vi "Stack_holderwise_total_bd_count_&_duration.vi"(0 "Refnum in":T1, 1 "BREAKDOWN_STK_HOLD_ID":i32=1, 2 "condition":string="Where BREAKDOWN_DATE between '%s'and '%s' and BREAKDOWN_STK_HOLD_ID ='%d'  ", 5 "Form Date":timestamp, 7 "Array":string[](array[string]), 9 "To Date":timestamp, 11 "error in (no error)":errorcluster, 12 "STATION_ID_CID_TRIGGER":i32, 13 "Shift":string(combo), 14 "tabel":string[](array[string])=["STATION_1_LOG_HISTORY", "STATION_2_LOG_HISTORY", "STATION_3_LOG_HISTORY", "STATION_4_LOG_HISTORY", "STATION_5_LOG_HISTORY", "STATION_6_LOG_HISTORY"]) -> (4 "Refnum out":T1, 6 "Count out":string[](array[string]), 10 "appended array":dbl[](array[numeric]), 15 "error out":errorcluster)   [LabVIEW 2017]
uses:
  <vilib>/addons/database/Connection.llb/Conn ObjectReference.ctl
  <vilib>/addons/database/NI_Database_API.lvlib
panel:
  out "Elements Found out":string[](array[string])
  out "Table":string[][](array[string])
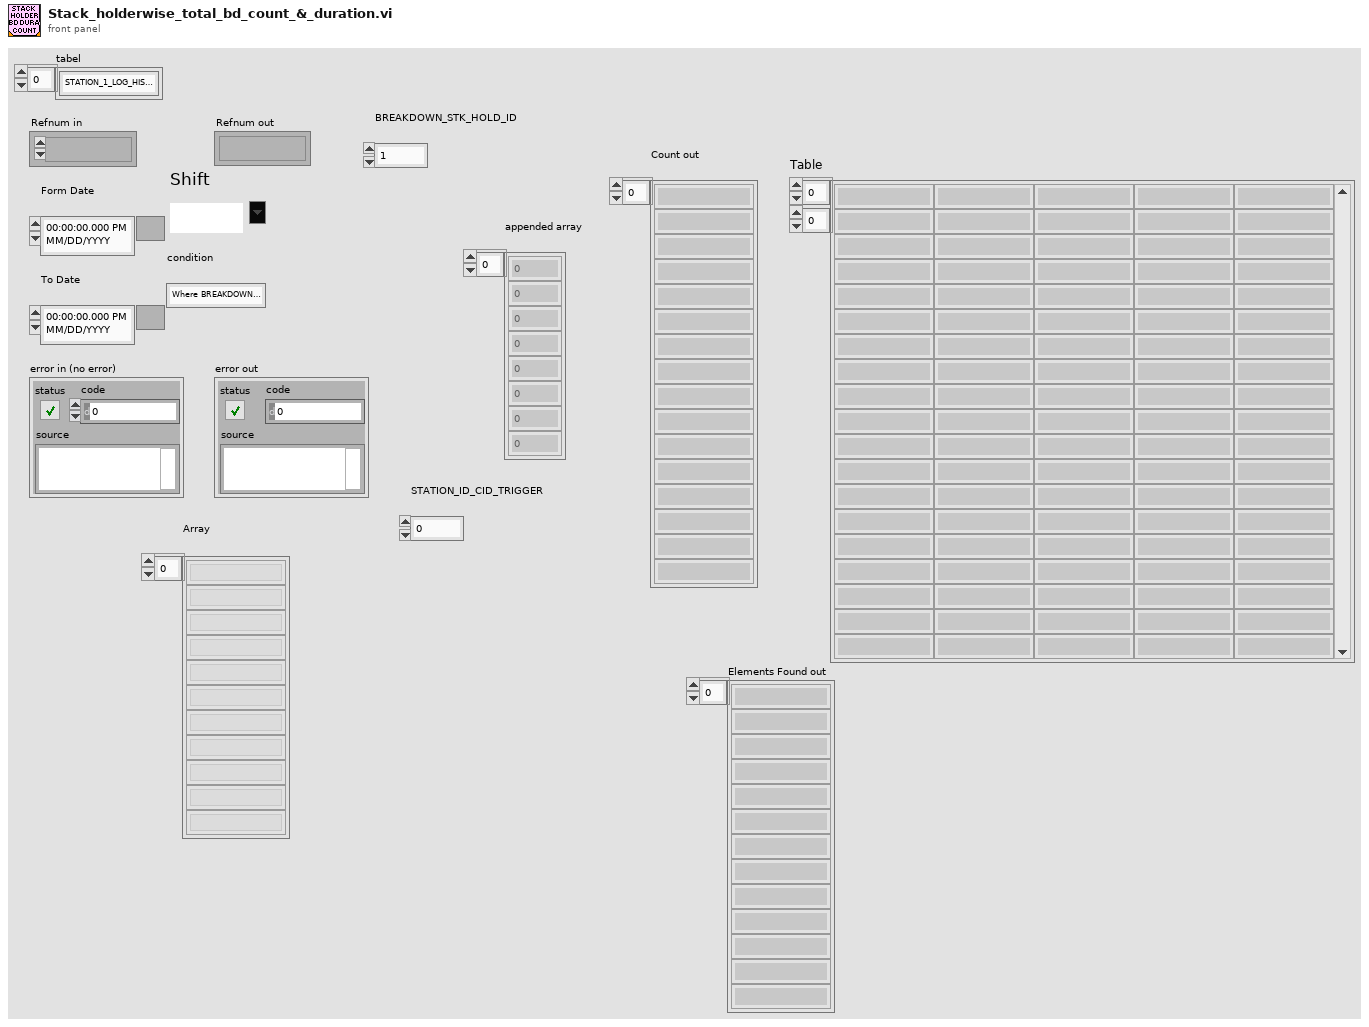
[diagram p1: front panel]
types:
  T1 = typedef "NI_Database_API.lvlib/Conn ObjectReference.ctl" = refnum<k1>
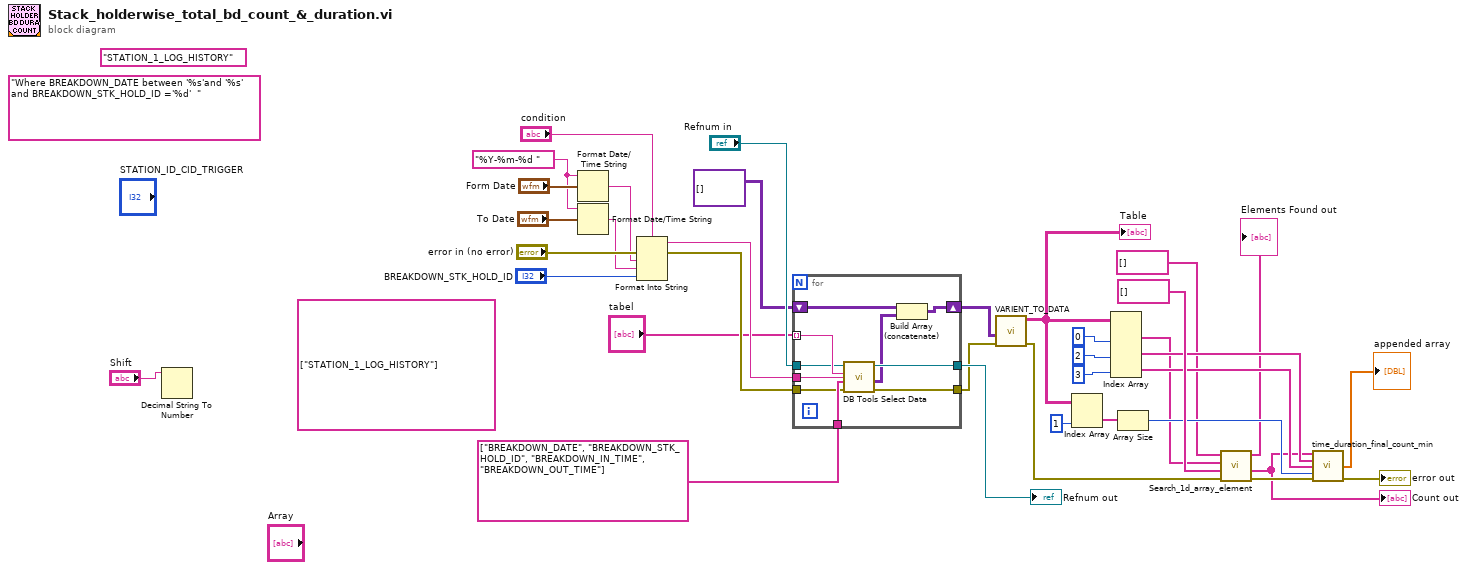
[diagram p0: block diagram]
diagram:
  (unwired) string[] ["STATION_1_LOG_HISTORY"]
  (unwired) "Where BREAKDOWN_DATE between '%s'and '%s' and BREAKDOWN_STK_HOLD_ID ='%d'  "
  (unwired) "STATION_1_LOG_HISTORY" ("table")
  w14 = "%Y-%m-%d " ("time format string (%c)")
  n1 = Decimal String To Number(string="Shift") -> ()  [unwired: 2 in, 2 out]
  n2 = Format Date/Time String(time format string (%c)=w14, seconds (now)="Form Date") -> (date/time string=w17:string)  [unwired: 1 in]
  n3 = Format Date/Time String(time format string (%c)=w14, seconds (now)="To Date") -> (date/time string=w18:string)  [unwired: 1 in]
  n4 = Format Into String(format string="condition", error in="error in (no error)", w17, w18, "BREAKDOWN_STK_HOLD_ID") -> (resulting string=w12:string, error out=w13:errorcluster)  [unwired: 1 in]
  n5 = for {
    tunnel: "tabel" -> [w46] mode=indexing
    tunnel: string[] ["BREAKDOWN_DATE", "BREAKDOWN_STK_HOLD_ID", "BREAKDOWN_IN_TIME", "BREAKDOWN_OUT_TIME"] -> [w45]
    tunnel: w12 -> [w41]
    shift-right: [w38] -> w6
    shift-left: variant[][] [] -> [w40]
    tunnel: "Refnum in" -> [w43]
    tunnel: [w44] -> w21
    tunnel: w13 -> [w42]
    tunnel: [w37] -> w3
    n6 = call <vilib>:"DB Tools Select Data.vi"("condition"=w41, "error in (no error)"=w42, "columns"=w45, "table"=w46, "connection reference"=w43) -> ("error out"=w37:errorcluster, "data"=w39:variant[][], "connection reference out"=w44:T1)  [unwired: 1 in]
    n7 = Build Array (concatenate)(w40, w39) -> (w38:variant[][])
  }
  "Refnum out" <- w21
  n8 = call "VARIENT_TO_DATA.vi"("data"=w6, "error in (no error)"=w3) -> ("Table"=w5:string[][], "error out"=w4:errorcluster)  [unwired: 7 in]
  "Table" <- w5
  n9 = Index Array(array=w5, index (col)=1 ("disabled index (col)")) -> (element=w28:string[])  [unwired: 1 in]
  n10 = Index Array(array=w5, index (col) #1=0 ("disabled index (col)"), index (col) #2=2 ("disabled index (col)"), index (col) #3=3 ("disabled index (col)")) -> (element #1=w30:string[], element #2=w32:string[], element #3=w33:string[])  [unwired: 3 in]
  n11 = Array Size(array=w28) -> (size(s)=w34:i32)
  n12 = call "Search_1d_array_element.vi"("error in (no error)"=w4, "Count in"=string[] [] ("Count"), "BD Date"=w30, "Elements Found in"=string[] [] ("Elements Found")) -> ("error out"=w31:errorcluster, "Count out"=w11:string[], "Elements Found out"=→"Elements Found out":string[])  [unwired: 3 in]
  "Count out" <- w11
  n13 = call "time_duration_final_count_min.vi"("BD Count"=w11, "Intime"=w32, "OutTime"=w33, "bd array size"=w34, "error in (no error)"=w31) -> ("appended array"=→"appended array":dbl[], "error out"=→"error out":errorcluster)  [unwired: 7 in, 2 out]
